vi "Programma.vi"() -> ()   [LabVIEW 2013]
panel:
  out "x = y?":bool
  in  "communicatie ?":bool=TRUE
  out "data out":string
  out "LifeForm 2":u32[][](array[colorbox])
  out "T button?":bool
  in  "Enum 2":enum16{"schrijf", "lees"}(ring)
  in  "eigen tekst":string
  in  "Eigen":bool[][](array[boolean])
  in  "Grootte":u32=20
  in  "milliseconds to wait":u32
  in  "Keuze":T1(ring)
  out "LifeForm":u32[][](array[colorbox])
  in  "Create Life uit keuze menu":bool
  # "Via keuze kan je data in de array sturen:\ninit, niks , communicatie en next versturen geen data."
  # "In het programma ( niet als server )\nAls je de eigen keuze kiest, kan je zelf iets tekenen in de eigen array OF je kan tekst tot maximum 20 tekens in de eigen tekst input typen\nDe eigen keuze geeft de optie voor het algoritme of weergeven\nAls je op weergeven duwt kan je niet switchen naar het algortime ! ( moet je het programma uitzetten en opnieuw opzetten)\nals server  via de client gaat dit wel ! ( door gewoon nieuwe data te versturen )"
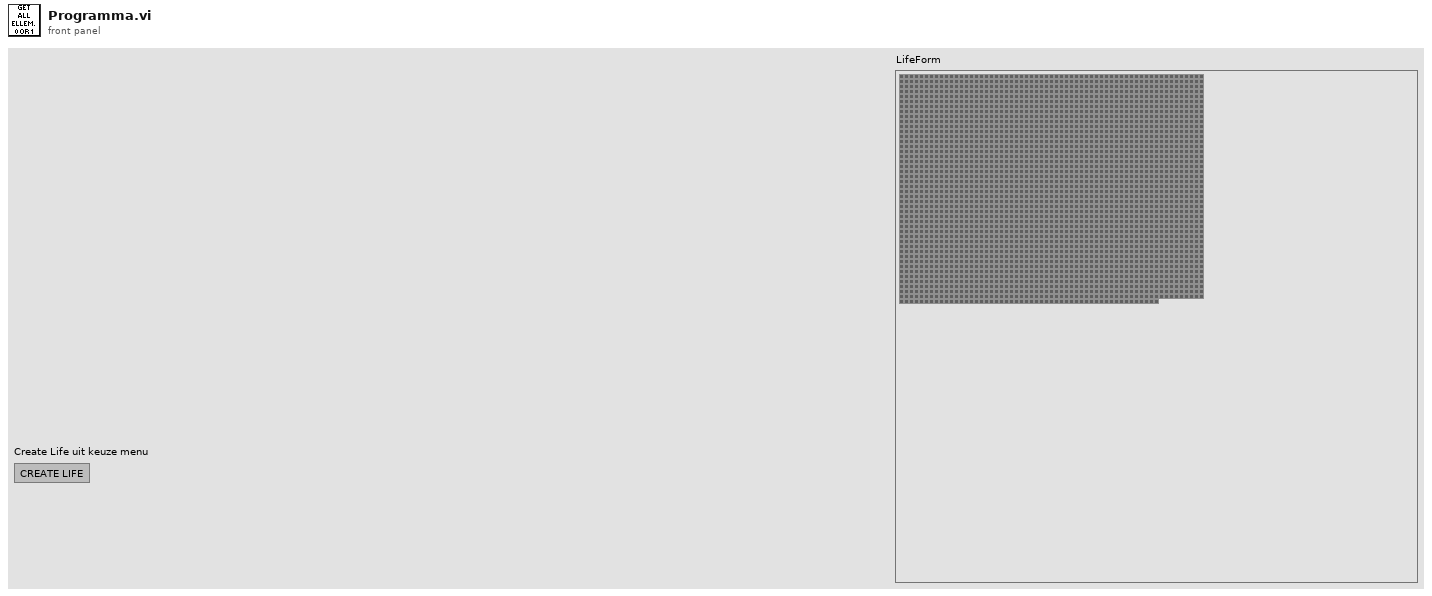
[diagram p1: front panel]
types:
  T1 = enum16{"Init", "Blinker", "Glider", "Block", "Next", "Toad", "Beehive", "Beacon", "Pulsar", "Eigen", "LWSS", "Niks", "Communicatie"}
  T2 = enum16{"Init", "Blinker", "Glider", "Block", "Next", "Toad", "Beehive", "Beacon", "Pulsar", "Eigen", "LWSS", "Niks", "Communicatie", "Lees"}
  T3 = enum16{"Init", "Blinker", "Glider", "Block", "Next"}
  T4 = enum16{"Init", "Blinker", "Glider", "Block", "Next", "Toad", "Beehive", "Beacon", "Pulsar", "Eigen", "LWSS"}
  T5 = enum16{"Init", "Blinker", "Glider", "Block", "Next", "Toad", "Beehive", "Beacon", "Pulsar", "Eigen", "LWSS", "Niks"}
  T6 = enum16{"Init", "Blinker", "Glider", "Block", "Next", "Toad"}
  T7 = enum16{"Init", "Blinker", "Glider", "Block", "Next", "Toad", "Beehive"}
  T8 = enum16{"Init", "Blinker", "Glider", "Block", "Next", "Toad", "Beehive", "Beacon"}
  T9 = enum16{"Init", "Blinker", "Glider", "Block", "Next", "Toad", "Beehive", "Beacon", "Pulsar"}
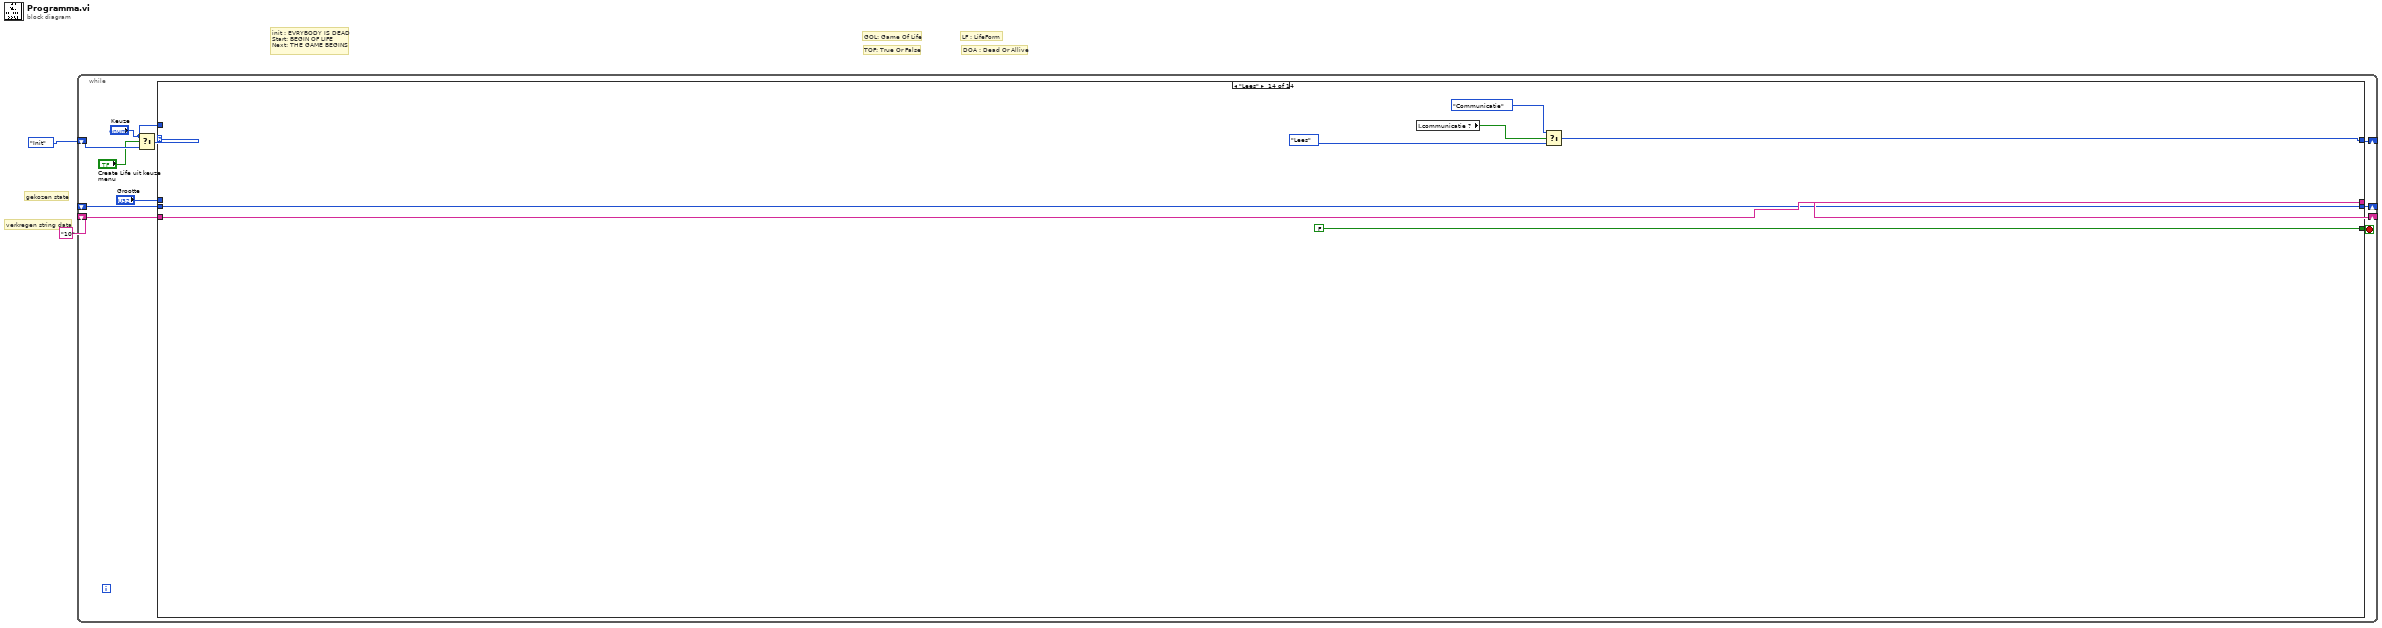
[diagram p0: block diagram]
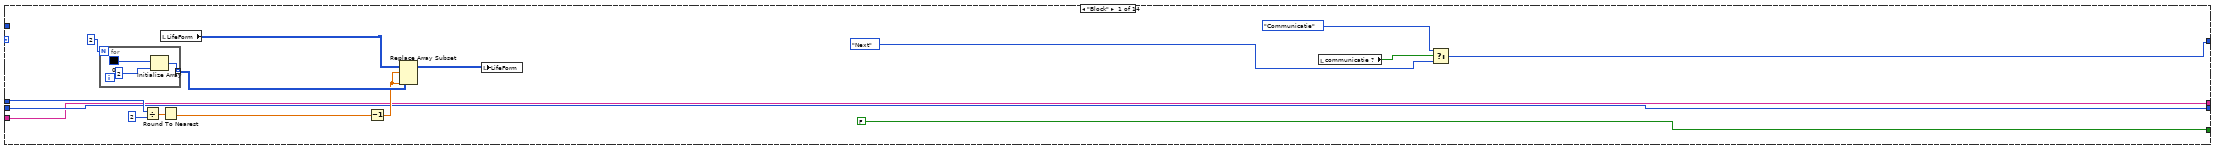
[diagram p2: hidden frame]
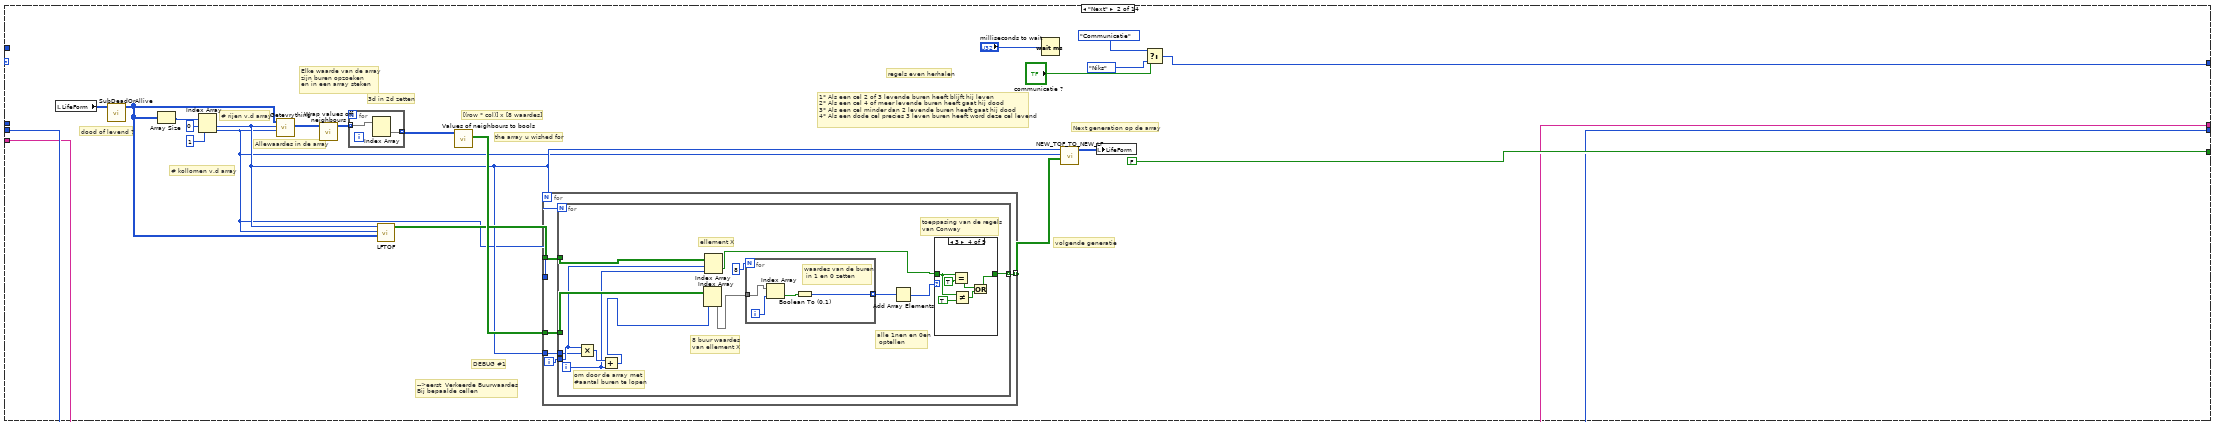
[diagram p3: hidden frame]
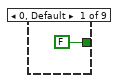
[diagram p4: hidden frame]
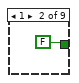
[diagram p5: hidden frame]
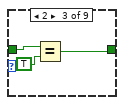
[diagram p6: hidden frame]
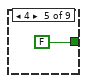
[diagram p7: hidden frame]
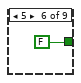
[diagram p8: hidden frame]
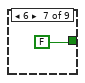
[diagram p9: hidden frame]
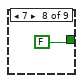
[diagram p10: hidden frame]
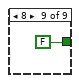
[diagram p11: hidden frame]
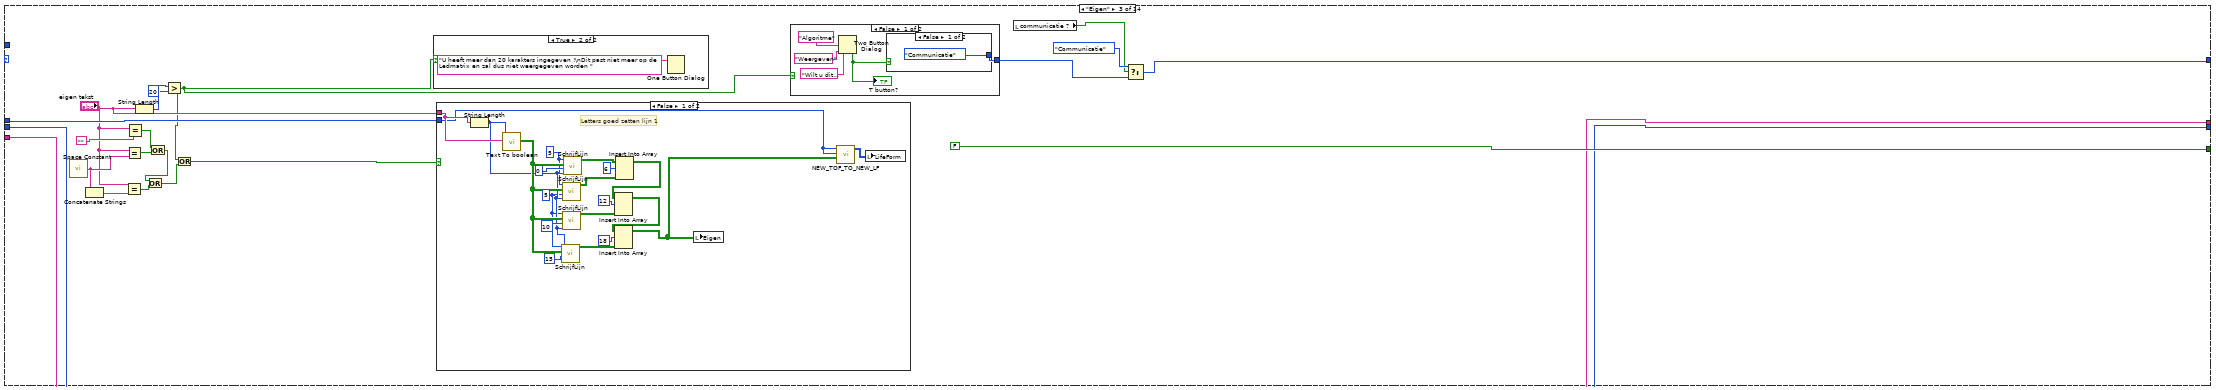
[diagram p12: hidden frame]
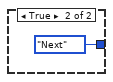
[diagram p13: hidden frame]
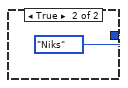
[diagram p14: hidden frame]
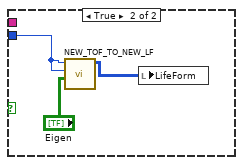
[diagram p16: hidden frame]
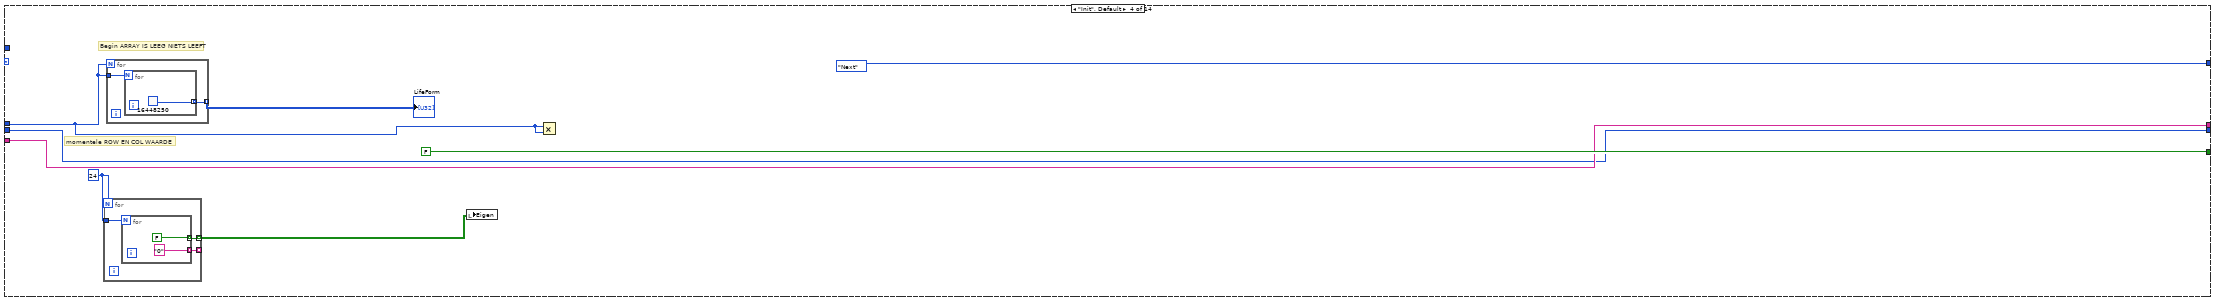
[diagram p17: hidden frame]
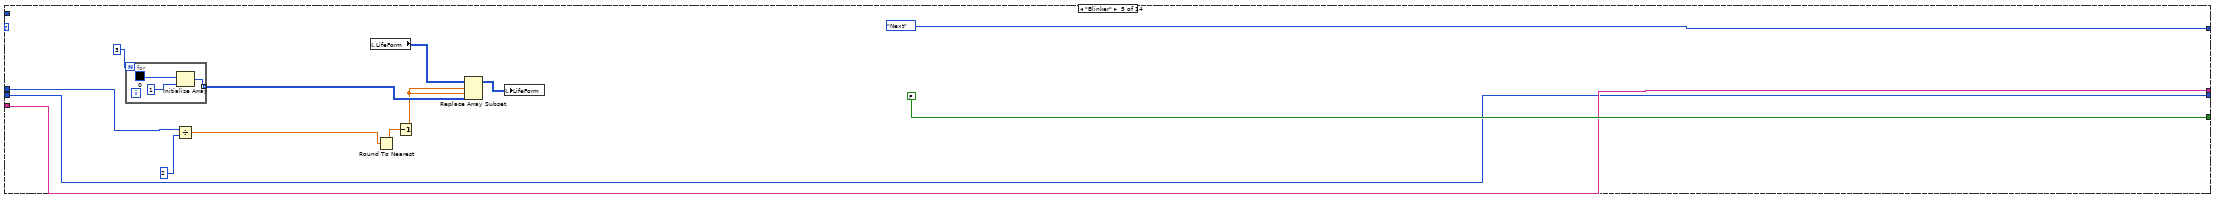
[diagram p18: hidden frame]
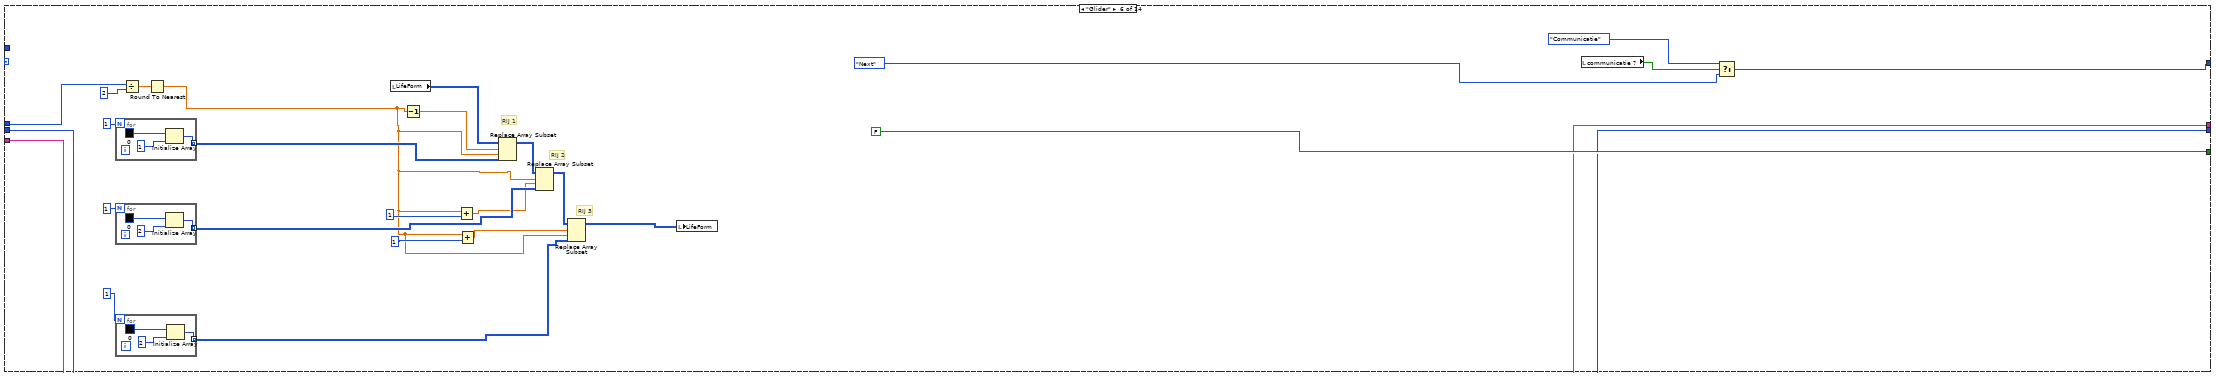
[diagram p19: hidden frame]
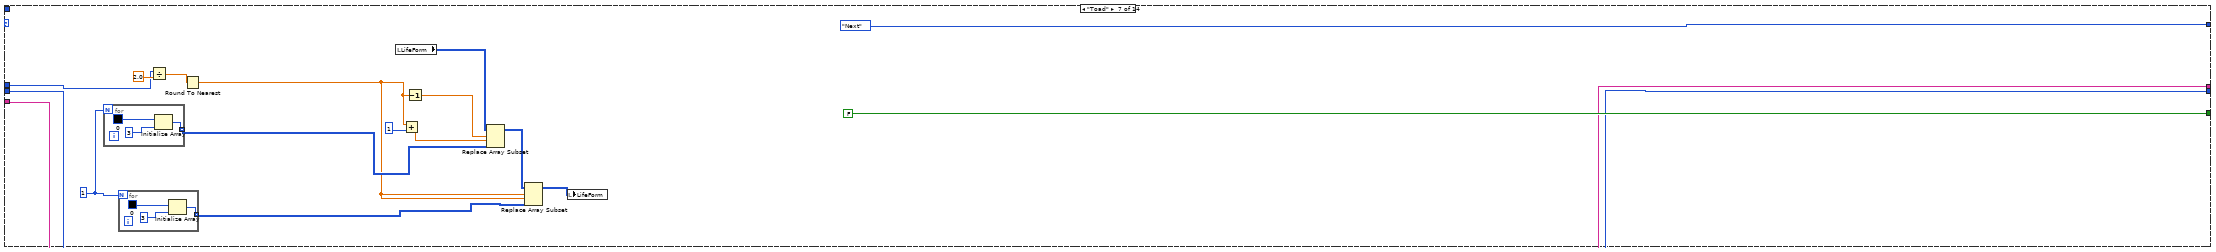
[diagram p20: hidden frame]
diagram:
  # "gekozen state"
  # "verkregen string data"
  # "DOA : Dead Or Allive"
  # "LF : LifeForm"
  # "TOF: True Or False"
  # "GOL: Game Of Life"
  # "init : EVRYBODY IS DEAD\nStart: BEGIN OF LIFE\nNext: THE GAME BEGINS"
  n1 = while {
    shift-right: [w12] -> _
    shift-left: T1."Init" ("Keuze") -> [w10]
    shift-right: [w7] -> _
    shift-left: "10" ("data out") -> [w6]
    shift-right: [w5] -> _
    shift-left: _ -> [w4]
    stop <- w13 stop-if-true
    n2 = Select(t="Keuze", s="Create Life uit keuze menu", f=w10) -> (s? t:f=w9:T2)
    n3 = case shown="\"Lees\"" w9 {
      tunnel: [FALSE FALSE FALSE FALSE FALSE FALSE FALSE FALSE FALSE FALSE FALSE FALSE w416 FALSE] -> w13
      tunnel: [w14 w38 w99 T3."Next" ("Enum") T3."Next" ("Enum") w182 T6."Next" ("Keuze") T7."Next" ("Keuze") T8."Next" ("Keuze") w284 w358 w395 w412 w497] -> w12
      tunnel: "Grootte" -> [w24 _ w116 w153 w171 w195 w225 w255 w275 w346 w371 _ w411 _]
      tunnel: "Keuze" -> [_ _ _ _ _ _ _ _ _ _ _ w400 _ _]
      tunnel: [w18 w33 w101 w150 w166 w186 w217 w240 w267 w289 w363 w402 w415 w502] -> w7
      tunnel: w6 -> [w18 w33 w101 w150 w166 w186 w217 w240 w267 w289 w363 w402 w410 w502]
      tunnel: [w19 w34 w100 w149 w165 w185 w216 w239 w266 w288 w362 w401 w412 w501] -> w5
      tunnel: w4 -> [w19 w34 w100 w149 w165 w185 w216 w239 w266 w288 w362 w401 w413 w501]
      frame "Block" {
        n4 = for {
          N: 2 -> [_]
          tunnel: [w30] -> w26 mode=indexing
          n5 = Initialize Array(u32 0 ("Color Box"), 2 ("dimension size")) -> (w30:u32[])
        }
        n6 = Divide(x=w24, y=u32 2) -> (x/y=w22:dbl)
        n7 = local read "LifeForm"() -> (w27:u32[][])
        n8 = Round To Nearest(number=w22) -> (nearest integer value=w21:dbl)
        n9 = Decrement(x=w21) -> (x-1=w20:dbl)
        n10 = Replace Array Subset(array=w27, new element=w26, index (row)=w20, index (col)=w20) -> (w25:u32[][])
        n11 = local write "LifeForm"(w25) -> ()
        n12 = local read "communicatie ?"() -> (w17:bool)
        n13 = Select(t=T2."Communicatie" ("Keuze"), s=w17, f=T3."Next" ("Enum")) -> (s? t:f=w14:T2)
      }
      frame "Next" {
        # "volgende generatie"
        # "regels even herhalen"
        # "Next generation op de array"
        # "Elke waarde van de array \nzijn buren opzoeken \nen in een array steken"
        # "-->eerst  Verkeerde Buurwaardes\nBij bepaalde cellen"
        # "dood of levend ?"
        # "Allewaardes in de array"
        # "DEBUG #1"
        # "1* Als een cel 2 of 3 levende buren heeft blijft hij leven\n2* Als een cel 4 of meer levende buren heeft gaat hij dood\n3* Als een cel minder dan 2 levende buren heeft gaat hij dood\n4* Als een dode cel precies 3 leven buren heeft word deze cel levend"
        # "[(row * col)] x [8 waardes]"
        # "# kollomen v.d array"
        # "# rijen v.d array"
        # "the array u wished for"
        # "3d in 2d zetten"
        n14 = local read "LifeForm"() -> (w44:u32[][])
        n15 = call "SubDeadOrAllive.vi"("Array"=w44) -> ("Array Dead Or Allive"=w48:u32[][])  [unwired: 10 in]
        n16 = Array Size(array=w48) -> (size(s)=w54:i32[])
        n17 = Index Array(array=w54, index #1=0 ("index"), index #2=1 ("index")) -> (element #1=w41:i32, element #2=w40:i32)
        n18 = call "Getevrything.vi"("Col"=w40, "Row"=w41, "Array Dead Or Allive"=w48) -> ("Array"=w51:u32[][][])  [unwired: 7 in, 1 out]
        n19 = call "Wrap values off neighbours.vi"("Array in"=w51) -> ("Array out"=w50:u32[][][])  [unwired: 10 in]
        n20 = for {
          tunnel: w50 -> [w95] mode=indexing
          tunnel: [w94] -> w49 mode=indexing
          n21 = Index Array(array=w95) -> (element=w94:u32[])  [unwired: 2 in]
        }
        n22 = call "LFTOF.vi"("LF DOA"=w48, "Col"=w40, "Row"=w41) -> ("LF TOF"=w46:bool[][])  [unwired: 8 in]
        n23 = call "Values of neighbours to bools.vi"("Array in"=w49) -> ("Array"=w47:bool[][])  [unwired: 9 in, 1 out]
        n24 = for {
          N: w41 -> [_]
          tunnel: w40 -> [w60]
          tunnel: w47 -> [w59]
          tunnel: w46 -> [w57]
          tunnel: [w56] -> w42 mode=indexing
          tunnel: w41 -> [w55]
          i -> [w58]
          # "om door de array met\n#aantal buren te lopen"
          n25 = for {
            N: w60 -> [_]
            tunnel: w59 -> [w73]
            tunnel: w58 -> [w68]
            tunnel: w57 -> [w70]
            tunnel: [w63] -> w56 mode=indexing
            tunnel: w55 -> [w61]
            i -> [w69]
            # "toeppasing van de regels\nvan Conway"
            # "alle 1nen en 0en\n optellen"
            # "ellement X"
            # "8 buur waardes\nvan ellement X"
            n26 = Multiply(x=w68, y=w61) -> (x*y=w72:i32)
            n27 = Add(x=w72, y=w69) -> (x+y=w71:i32)
            n28 = Index Array(array=w73, index (row)=w71) -> (element=w64:bool[])  [unwired: 1 in]
            n29 = Index Array(array=w70, index (row)=w68, index (col)=w69) -> (element=w65:bool)
            n30 = for {
              N: 8 -> [_]
              tunnel: w64 -> [w93]
              tunnel: [w90] -> w66 mode=indexing
              i -> [w92]
              # "waardes van de buren\n in 1 en 0 zetten"
              n31 = Index Array(array=w93, index=w92) -> (element=w91:bool)
              n32 = Boolean To (0,1)(Boolean=w91) -> (0, 1=w90:i16)
            }
            n33 = Add Array Elements(numeric array=w66) -> (sum=w62:i16)
            n34 = case shown="3" w62 {
              tunnel: w65 -> [_ _ w78 w83 _ _ _ _ _]
              tunnel: [FALSE FALSE w76 w79 FALSE FALSE FALSE FALSE FALSE] -> w63
              frame 0, Default {
              }
              frame 1 {
              }
              frame 2 {
                n35 = Equal?(x=w78, y=TRUE) -> (x = y?=w76:bool)
              }
              frame 3 {
                n36 = Equal?(x=w83, y=TRUE) -> (x = y?=w80:bool)
                n37 = Not Equal?(x=w83, y=TRUE) -> (x != y?=w81:bool)
                n38 = Or(x=w80, y=w81) -> (x .or. y?=w79:bool)
              }
              frame 4 {
              }
              frame 5 {
              }
              frame 6 {
              }
              frame 7 {
              }
              frame 8 {
              }
            }
          }
        }
        n39 = Wait (ms)(milliseconds to wait="milliseconds to wait") -> ()  [unwired: 1 out]
        n40 = call "NEW_TOF_TO_NEW_LF.vi"("NEXT TOF"=w42, "Col"=w40, "Row"=w41) -> ("Next LF"=w39:u32[][])  [unwired: 8 in]
        n41 = local write "LifeForm"(w39) -> ()
        n42 = Select(t=T2."Communicatie" ("Keuze"), s="communicatie ?", f=T2."Niks" ("Keuze")) -> (s? t:f=w38:T2)
      }
      frame "Eigen" {
        n43 = call <vilib>:"Space Constant.vi"() -> ("String"=w111:string)
        n44 = Concatenate Strings(w111, w111) -> (w110:string)
        n45 = Equal?(x="eigen tekst", y=w110) -> (x = y?=w109:bool)
        n46 = Equal?(x="eigen tekst", y=w111) -> (x = y?=w112:bool)
        n47 = Equal?(x="eigen tekst", y="") -> (x = y?=w113:bool)
        n48 = String Length(string="eigen tekst") -> (length=w106:i32)
        n49 = Or(x=w113, y=w112) -> (x .or. y?=w108:bool)
        n50 = Or(x=w108, y=w109) -> (x .or. y?=w104:bool)
        n51 = Greater?(x=w106, y=20) -> (0:w102:bool)
        n52 = Or(x=w102, y=w104) -> (x .or. y?=w103:bool)
        n53 = case shown="True" w102 {
          frame False {
          }
          frame True {
            n54 = One Button Dialog(message="U heeft meer dan 20 karakters ingegeven !\nDit past niet meer op de Ledmatrix en zal dus niet weergegeven worden ") -> ()  [unwired: 1 in, 1 out]
          }
        }
        n55 = case shown="False" w103 {
          tunnel: w116 -> [w144 w148]
          tunnel: "eigen tekst" -> [w145 _]
          frame False {
            w126 = 5 ("x")
            w127 = 5
            # "Letters goed zetten lijn 1"
            n56 = String Length(string=w145) -> (length=w138:i32)
            n57 = call "Text To boolean.vi"("eigen tekst"=w145, "Numeric"=w138) -> ("Letter"=w140:bool[][][])  [unwired: 9 in]
            n58 = call "SchrijfLijn.vi"("Lengte"=w138, "x"=15, "Letter in"=w140, "Numeric"=w126) -> ("Letter out"=w129:bool[][])  [unwired: 7 in]
            n59 = call "SchrijfLijn.vi"("Lengte"=w138, "x"=w126, "Letter in"=w140, "Numeric"=w127) -> ("Letter out"=w135:bool[][])  [unwired: 7 in]
            n60 = call "SchrijfLijn.vi"("Lengte"=w138, "x"=10, "Letter in"=w140, "Numeric"=w126) -> ("Letter out"=w132:bool[][])  [unwired: 7 in]
            n61 = call "SchrijfLijn.vi"("Lengte"=w138, "x"=0, "Letter in"=w140, "Numeric"=w127) -> ("Letter out"=w137:bool[][])  [unwired: 7 in]
            n62 = Insert Into Array(array=w137, index (row)=6, new element=w135) -> (w133:bool[][])  [unwired: 1 in]
            n63 = Insert Into Array(array=w133, index (row)=12, new element=w132) -> (w131:bool[][])  [unwired: 1 in]
            n64 = Insert Into Array(array=w131, index (row)=18, new element=w129) -> (w128:bool[][])  [unwired: 1 in]
            n65 = local write "Eigen"(w128) -> ()
            n66 = call "NEW_TOF_TO_NEW_LF.vi"("NEXT TOF"=w128, "Col"=w144, "Row"=w144) -> ("Next LF"=w143:u32[][])  [unwired: 8 in]
            n67 = local write "LifeForm"(w143) -> ()
          }
          frame True {
            n68 = call "NEW_TOF_TO_NEW_LF.vi"("NEXT TOF"="Eigen", "Col"=w148, "Row"=w148) -> ("Next LF"=w146:u32[][])  [unwired: 8 in]
            n69 = local write "LifeForm"(w146) -> ()
          }
        }
        n70 = case shown="False" w102 {
          tunnel: [w120 T5."Niks" ("Keuze")] -> w98
          frame False {
            n71 = Two Button Dialog(message="Wilt u dit gewoon weergeven of wilt u  het algoritme hierop toepassen ?", 1:"Weergeven" ("F button name (\"Cancel\")"), 2:"Algoritme" ("T button name (\"OK\")")) -> (T button?=w119:bool)
            "T button?" <- w119
            n72 = case shown="False" w119 {
              tunnel: [T2."Communicatie" ("Keuze") T4."Next" ("Keuze")] -> w120
              frame False {
              }
              frame True {
              }
            }
          }
          frame True {
          }
        }
        n73 = local read "communicatie ?"() -> (w96:bool)
        n74 = Select(t=T2."Communicatie" ("Keuze"), s=w96, f=w98) -> (s? t:f=w99:T2)
      }
      frame "Init", Default {
        w152 = 24
        # "momentele ROW EN COL WAARDE"
        # "Begin ARRAY IS LEEG NIETS LEEFT"
        n75 = for {
          N: w152 -> [_]
          tunnel: w152 -> [w159]
          tunnel: [w158] -> w151 mode=indexing
          tunnel: [w157] -> _ mode=indexing
          n76 = for {
            N: w159 -> [_]
            tunnel: [FALSE] -> w158 mode=indexing
            tunnel: ["0"] -> w157 mode=indexing
          }
        }
        n77 = for {
          N: w153 -> [_]
          tunnel: w153 -> [w163]
          tunnel: [w162] -> w156 mode=indexing
          n78 = for {
            N: w163 -> [_]
            tunnel: [u32 16448250 ("Color Box")] -> w162 mode=indexing
          }
        }
        "LifeForm" <- w156
        n79 = local write "Eigen"(w151) -> ()
        n80 = Multiply(x=w153, y=w153) -> ()  [unwired: 1 out]
      }
      frame "Blinker" {
        n81 = for {
          N: 3 -> [_]
          tunnel: [w178] -> w176 mode=indexing
          n82 = Initialize Array(u32 0 ("Color Box"), 1 ("dimension size")) -> (w178:u32[])
        }
        n83 = Divide(x=w171, y=u32 2) -> (x/y=w170:dbl)
        n84 = local read "LifeForm"() -> (w174:u32[][])
        n85 = Round To Nearest(number=w170) -> (nearest integer value=w168:dbl)
        n86 = Decrement(x=w168) -> (x-1=w169:dbl)
        n87 = Replace Array Subset(array=w174, new element=w176, index (row)=w169, index (col)=w169) -> (w175:u32[][])
        n88 = local write "LifeForm"(w175) -> ()
      }
      frame "Glider" {
        # "RIJ 3"
        # "RIJ 2"
        # "RIJ 1"
        n89 = for {
          N: 1 -> [_]
          tunnel: [w213] -> w201 mode=indexing
          n90 = Initialize Array(u32 0 ("Color Box"), 1 ("dimension size")) -> (w213:u32[])
        }
        n91 = for {
          N: 1 -> [_]
          tunnel: [w210] -> w199 mode=indexing
          n92 = Initialize Array(u32 0 ("Color Box"), 2 ("dimension size")) -> (w210:u32[])
        }
        n93 = for {
          N: 1 -> [_]
          tunnel: [w207] -> w197 mode=indexing
          n94 = Initialize Array(u32 0 ("Color Box"), 2 ("dimension size")) -> (w207:u32[])
        }
        n95 = Divide(x=w195, y=u32 2) -> (x/y=w189:dbl)
        n96 = Round To Nearest(number=w189) -> (nearest integer value=w187:dbl)
        n97 = local read "LifeForm"() -> (w202:u32[][])
        n98 = Decrement(x=w187) -> (x-1=w188:dbl)
        n99 = Add(x=w187, y=1 ("disabled index (col)")) -> (x+y=w193:dbl)
        n100 = Add(x=w187, y=1 ("index (row)")) -> (x+y=w190:dbl)
        n101 = Replace Array Subset(array=w202, new element=w201, index (row)=w188, index (col)=w187) -> (w200:u32[][])
        n102 = Replace Array Subset(array=w200, new element=w199, index (row)=w187, index (col)=w193) -> (w198:u32[][])
        n103 = Replace Array Subset(array=w198, new element=w197, index (row)=w190, index (col)=w187) -> (w196:u32[][])
        n104 = local write "LifeForm"(w196) -> ()
        n105 = local read "communicatie ?"() -> (w181:bool)
        n106 = Select(t=T2."Communicatie" ("Keuze"), s=w181, f=T3."Next" ("Enum")) -> (s? t:f=w182:T2)
      }
      frame "Toad" {
        w218 = 1
        n107 = for {
          N: w218 -> [_]
          tunnel: [w236] -> w224 mode=indexing
          n108 = Initialize Array(u32 0 ("Color Box"), 3 ("dimension size")) -> (w236:u32[])
        }
        n109 = for {
          N: w218 -> [_]
          tunnel: [w233] -> w231 mode=indexing
          n110 = Initialize Array(u32 0 ("Color Box"), 3 ("dimension size")) -> (w233:u32[])
        }
        n111 = Divide(x=w225, y=2.0) -> (x/y=w221:dbl)
        n112 = Round To Nearest(number=w221) -> (nearest integer value=w219:dbl)
        n113 = local read "LifeForm"() -> (w229:u32[][])
        n114 = Add(x=w219, y=1 ("disabled index (col)")) -> (x+y=w222:dbl)
        n115 = Decrement(x=w219) -> (x-1=w220:dbl)
        n116 = Replace Array Subset(array=w229, new element=w224, index (row)=w220, index (col)=w222) -> (w232:u32[][])
        n117 = Replace Array Subset(array=w232, new element=w231, index (row)=w219, index (col)=w219) -> (w230:u32[][])
        n118 = local write "LifeForm"(w230) -> ()
      }
      frame "Beehive" {
        w251 = 1
        n119 = for {
          N: w251 -> [_]
          tunnel: [w263] -> w245 mode=indexing
          n120 = Initialize Array(u32 0 ("Color Box"), 2 ("dimension size")) -> (w263:u32[])
        }
        n121 = for {
          N: w251 -> [_]
          tunnel: [w260] -> w247 mode=indexing
          n122 = Initialize Array(u32 0 ("Color Box"), 1 ("dimension size")) -> (w260:u32[])
        }
        n123 = Divide(x=w255, y=2.0) -> (x/y=w257:dbl)
        n124 = Round To Nearest(number=w257) -> (nearest integer value=w242:dbl)
        n125 = local read "LifeForm"() -> (w256:u32[][])
        n126 = Increment(x=w242) -> (x+1=w241:dbl)
        n127 = Decrement(x=w242) -> (x-1=w244:dbl)
        n128 = Replace Array Subset(array=w256, new element=w245, index (row)=w244, index (col)=w241) -> (w259:u32[][])
        n129 = Increment(x=w242) -> (x+1=w243:dbl)
        n130 = Add(x=w242, y=2.0) -> (x+y=w249:dbl)
        n131 = Replace Array Subset(array=w259, new element=w247, index (row)=w242, index (col)=w242) -> (w250:u32[][])
        n132 = Replace Array Subset(array=w250, new element=w247, index (row)=w242, index (col)=w249) -> (w246:u32[][])
        n133 = Replace Array Subset(array=w246, new element=w245, index (row)=w243, index (col)=w243) -> (w254:u32[][])
        n134 = local write "LifeForm"(w254) -> ()
      }
      frame "Beacon" {
        n135 = for {
          N: 2 -> [_]
          tunnel: [w281] -> w274 mode=indexing
          n136 = Initialize Array(u32 0 ("Color Box"), 2 ("dimension size")) -> (w281:u32[])
        }
        n137 = local read "LifeForm"() -> (w276:u32[][])
        n138 = Divide(x=w275, y=u32 2) -> (x/y=w278:dbl)
        n139 = Round To Nearest(number=w278) -> (nearest integer value=w273:dbl)
        n140 = Decrement(x=w273) -> (x-1=w277:dbl)
        n141 = Increment(x=w273) -> (x+1=w271:dbl)
        n142 = Replace Array Subset(array=w276, new element=w274, index (row)=w277, index (col)=w277) -> (w270:u32[][])
        n143 = Replace Array Subset(array=w270, new element=w274, index (row)=w271, index (col)=w271) -> (w272:u32[][])
        n144 = local write "LifeForm"(w272) -> ()
      }
      frame "Pulsar" {
        # "Horizontaal 4"
        # "VERTICAAL 2"
        # "Horizontaal 3"
        # "Horizontaal 2"
        # "Verticaal 1"
        # "Horizontaal 3"
        # "Horizontaal 1"
        n145 = for {
          N: 3 -> [_]
          tunnel: [w352] -> w301 mode=indexing
          n146 = Initialize Array(u32 0 ("Color Box"), 1 ("dimension size")) -> (w352:u32[])
        }
        n147 = for {
          N: 1 -> [_]
          tunnel: [w355] -> w294 mode=indexing
          n148 = Initialize Array(u32 0 ("Color Box"), 3 ("dimension size")) -> (w355:u32[])
        }
        n149 = Divide(x=w346, y=u32 2) -> (x/y=w348:dbl)
        n150 = Round To Nearest(number=w348) -> (nearest integer value=w291:dbl)
        n151 = local read "LifeForm"() -> (w336:u32[][])
        n152 = Subtract(x=w291, y=6.0) -> (x-y=w343:dbl)
        n153 = Add(x=w291, y=2.0) -> (x+y=w342:dbl)
        n154 = Subtract(x=w291, y=4.0) -> (x-y=w327:dbl)
        n155 = Subtract(x=w291, y=6.0) -> (x-y=w338:dbl)
        n156 = Subtract(x=w291, y=4.0) -> (x-y=w344:dbl)
        n157 = Decrement(x=w291) -> (x-1=w332:dbl)
        n158 = Increment(x=w291) -> (x+1=w330:dbl)
        n159 = Add(x=w291, y=6.0) -> (x+y=w326:dbl)
        n160 = Replace Array Subset(array=w336, new element=w294, index (row)=w343, index (col)=w344) -> (w335:u32[][])
        n161 = Replace Array Subset(array=w335, new element=w294, index (row)=w343, index (col)=w342) -> (w334:u32[][])
        n162 = Replace Array Subset(array=w334, new element=w301, index (row)=w327, index (col)=w338) -> (w333:u32[][])
        n163 = Replace Array Subset(array=w333, new element=w301, index (row)=w327, index (col)=w332) -> (w331:u32[][])
        n164 = Replace Array Subset(array=w331, new element=w301, index (row)=w327, index (col)=w330) -> (w329:u32[][])
        n165 = Replace Array Subset(array=w329, new element=w301, index (row)=w327, index (col)=w326) -> (w323:u32[][])
        n166 = Subtract(x=w291, y=6.0) -> (x-y=w307:dbl)
        n167 = Decrement(x=w291) -> (x-1=w305:dbl)
        n168 = Add(x=w291, y=6.0) -> (x+y=w302:dbl)
        n169 = Increment(x=w291) -> (x+1=w318:dbl)
        n170 = Increment(x=w291) -> (x+1=w304:dbl)
        n171 = Subtract(x=w291, y=4.0) -> (x-y=w314:dbl)
        n172 = Decrement(x=w291) -> (x-1=w319:dbl)
        n173 = Add(x=w291, y=2.0) -> (x+y=w306:dbl)
        n174 = Subtract(x=w291, y=4.0) -> (x-y=w320:dbl)
        n175 = Add(x=w291, y=2.0) -> (x+y=w322:dbl)
        n176 = Replace Array Subset(array=w323, new element=w294, index (row)=w319, index (col)=w320) -> (w321:u32[][])
        n177 = Replace Array Subset(array=w321, new element=w294, index (row)=w319, index (col)=w322) -> (w317:u32[][])
        n178 = Replace Array Subset(array=w317, new element=w294, index (row)=w318, index (col)=w314) -> (w316:u32[][])
        n179 = Replace Array Subset(array=w316, new element=w294, index (row)=w318, index (col)=w306) -> (w309:u32[][])
        n180 = Replace Array Subset(array=w309, new element=w301, index (row)=w306, index (col)=w307) -> (w312:u32[][])
        n181 = Replace Array Subset(array=w312, new element=w301, index (row)=w306, index (col)=w305) -> (w311:u32[][])
        n182 = Replace Array Subset(array=w311, new element=w301, index (row)=w306, index (col)=w304) -> (w310:u32[][])
        n183 = Replace Array Subset(array=w310, new element=w301, index (row)=w306, index (col)=w302) -> (w300:u32[][])
        n184 = Add(x=w291, y=6.0) -> (x+y=w293:dbl)
        n185 = Subtract(x=w291, y=4.0) -> (x-y=w295:dbl)
        n186 = Add(x=w291, y=2.0) -> (x+y=w290:dbl)
        n187 = Replace Array Subset(array=w300, new element=w294, index (row)=w293, index (col)=w295) -> (w298:u32[][])
        n188 = Replace Array Subset(array=w298, new element=w294, index (row)=w293, index (col)=w290) -> (w299:u32[][])
        n189 = local write "LifeForm"(w299) -> ()
        n190 = local read "communicatie ?"() -> (w285:bool)
        n191 = Select(t=T2."Communicatie" ("Keuze"), s=w285, f=T9."Next" ("Keuze")) -> (s? t:f=w284:T2)
      }
      frame "LWSS" {
        n192 = for {
          N: 1 -> [_]
          tunnel: [w389] -> w372 mode=indexing
          n193 = Initialize Array(u32 0 ("Color Box"), 4 ("dimension size")) -> (w389:u32[])
        }
        n194 = Divide(x=w371, y=u32 2) -> (x/y=w387:dbl)
        n195 = for {
          N: 1 -> [_]
          tunnel: [w392] -> w369 mode=indexing
          n196 = Initialize Array(u32 0 ("Color Box"), 2 ("dimension size")) -> (w392:u32[])
        }
        n197 = Round To Nearest(number=w387) -> (nearest integer value=w386:dbl)
        n198 = Decrement(x=w386) -> (x-1=w366:dbl)
        n199 = local read "LifeForm"() -> (w384:u32[][])
        n200 = Decrement(x=w366) -> (x-1=w365:dbl)
        n201 = Subtract(x=w366, y=2.0) -> (x-y=w380:dbl)
        n202 = Subtract(x=w366, y=2.0) -> (x-y=w374:dbl)
        n203 = Increment(x=w366) -> (x+1=w378:dbl)
        n204 = Increment(x=w366) -> (x+1=w376:dbl)
        n205 = Increment(x=w376) -> (x+1=w368:dbl)
        n206 = Increment(x=w368) -> (x+1=w367:dbl)
        n207 = Replace Array Subset(array=w384, new element=w369, index (row)=w366, index (col)=w366) -> (w382:u32[][])
        n208 = Replace Array Subset(array=w382, new element=w369, index (row)=w376, index (col)=w380) -> (w379:u32[][])
        n209 = Replace Array Subset(array=w379, new element=w369, index (row)=w376, index (col)=w378) -> (w377:u32[][])
        n210 = Replace Array Subset(array=w377, new element=w372, index (row)=w368, index (col)=w374) -> (w370:u32[][])
        n211 = Replace Array Subset(array=w370, new element=w369, index (row)=w367, index (col)=w365) -> (w364:u32[][])
        n212 = local write "LifeForm"(w364) -> ()
        n213 = local read "communicatie ?"() -> (w359:bool)
        n214 = Select(t=T2."Communicatie" ("Keuze"), s=w359, f=T4."Next" ("Keuze")) -> (s? t:f=w358:T2)
      }
      frame "Niks" {
        w396 = T2."Next" ("Keuze")
        n215 = local read "communicatie ?"() -> (w397:bool)
        n216 = Select(t=T2."Communicatie" ("Keuze"), s=w397, f=w400) -> (s? t:f=w399:T2)
        n217 = local read "T button?"() -> (w404:bool)
        n218 = Not Equal?(x=w399, y=T2."Eigen" ("Keuze")) -> (x != y?=w406:bool)
        n219 = Select(t=w396, s=w406, f=T2."Lees" ("Keuze")) -> (s? t:f=w403:T2)
        n220 = Select(t=w396, s=w404, f=w403) -> (s? t:f=w395:T2)
      }
      frame "Communicatie" {
        # "0 : kies vanuit programma\n1: block\n2: custom\n3: glider \n4: Pulsar\n5: LWSS\n6: init ( leegmaken )"
        # "An IPv4 packet is limited to a size of 65,535 bytes. However the lower layers of a TCP/IP connection typically have lower packet sizes: I.e. the \"Maximum Transmission Unit\" (MTU) for Ethernet is around 1,500 bytes.\nBandwith consideration\nBe aware that the bandwidth of a TCP/IP connection is limited. A 500,000-element array of type DBL like described in the issue above equals approximately 4MB of user data. Transferring this array three times per second already oversaturates a 100MBit/s Fast Ethernet connection."
        # "deze waardes in 1 string zetten"
        # "de hele lifeform nakijken en de waardes omzetten in 1 of 0"
        n221 = call <vilib>:"TCP Listen.vi"("port"=u16 20, "service name"="localhost") -> ("error out"=w429:errorcluster, "connection ID"=w430:refnum<k5>)  [unwired: 5 in, 3 out]
        n222 = TCP Read(connection ID=w430, bytes to read=1, error in (no error)=w429) -> (connection ID out=w423:refnum<k5>, data out=w414:string, error out=w425:errorcluster)  [unwired: 2 in]
        "data out" <- w414
        n223 = Number To Decimal String(number=w411) -> (decimal integer string=w421:string)  [unwired: 1 in]
        n224 = local read "LifeForm"() -> (w428:u32[][])
        n225 = TCP Write(connection ID=w423, data in=w421, error in (no error)=w425) -> (connection ID out=w422:refnum<k5>, error out=w424:errorcluster)  [unwired: 1 in, 1 out]
        n226 = for {
          N: w411 -> [_]
          tunnel: w428 -> [w482]
          tunnel: w411 -> [w476]
          tunnel: w422 -> [w481]
          tunnel: w424 -> [w480]
          tunnel: [w479] -> w420
          tunnel: [w478] -> w419
          i -> [w477]
          n227 = for {
            N: w476 -> [_]
            tunnel: w482 -> [w496]
            tunnel: w477 -> [w495]
            tunnel: w481 -> [w489]
            tunnel: w480 -> [w488]
            tunnel: [w487] -> w479
            tunnel: [w486] -> w478
            i -> [w484]
            # "je begint op 0 dus +1"
            # "WIT"
            n228 = Index Array(array=w496, index (row)=w495, index (col)=w484) -> (element=w494:u32)
            n229 = Equal?(x=w494, y=u32 16448250) -> (x = y?=w492:bool)
            n230 = Select(t=0.0, s=w492, f=1.0) -> (s? t:f=w490:dbl)
            n231 = Number To Decimal String(number=w490) -> (decimal integer string=w483:string)  [unwired: 1 in]
            n232 = TCP Write(connection ID=w489, data in=w483, error in (no error)=w488) -> (connection ID out=w487:refnum<k5>, error out=w486:errorcluster)  [unwired: 1 in, 1 out]
          }
        }
        n233 = case shown="No Error" w419 {
          tunnel: w420 -> [w474 _]
          tunnel: w419 -> [w473 _]
          tunnel: [FALSE ("abort (F)") TRUE ("abort (F)")] -> w417
          frame No Error {
            n234 = TCP Close Connection(connection ID=w474, error in (no error)=w473) -> ()  [unwired: 1 in, 2 out]
          }
          frame Error {
          }
        }
        n235 = Equal?(x=w414, y=w410) -> (x = y?=w409:bool)
        "x = y?" <- w409
        n236 = case shown="True" w409 {
          selector: w409 -> [w433 _]
          tunnel: [w432 w455] -> w412
          tunnel: [w434 w456] -> w415
          tunnel: w414 -> [w435 w456]
          tunnel: w413 -> [_ w457]
          frame False {
            n237 = case shown="\"7\"" w435 {
              selector: w435 -> [w436 w439 w440 w442 w445 w446 w449 w450]
              tunnel: [T2."Block" ("Keuze") T2."Eigen" ("Keuze") T2."Glider" ("Keuze") T2."Pulsar" ("Keuze") T2."LWSS" ("Keuze") T2."Init" ("Keuze") T2."Niks" ("Keuze") w451] -> w432
              tunnel: [w436 w439 w440 w442 w445 w446 w449 w450] -> w434
              tunnel: w433 -> [_ _ _ _ _ _ _ _]
              frame "1" {
              }
              frame "2" {
              }
              frame "3" {
              }
              frame "4" {
              }
              frame "5" {
              }
              frame "6" {
                # "Begin ARRAY IS LEEG NIETS LEEFT"
              }
              frame "0", Default {
              }
              frame "7" {
                n238 = local read "T button?"() -> (w454:bool)
                n239 = Select(t=T2."Niks" ("Keuze"), s=w454, f=T2."Lees" ("Keuze")) -> (s? t:f=w451:T2)
              }
            }
          }
          frame True {
            n240 = case shown="\"1\", Default" w456 {
              tunnel: w457 -> [_ _ _ _ _ _ _ _]
              tunnel: [T2."Niks" ("Keuze") T2."Niks" ("Keuze") w463 T2."Niks" ("Keuze") T2."Niks" ("Keuze") T2."Niks" ("Keuze") T2."Niks" ("Keuze") w468] -> w455
              frame "1", Default {
              }
              frame "0" {
              }
              frame "2" {
                n241 = local read "T button?"() -> (w462:bool)
                n242 = Select(t=T2."Niks" ("Keuze"), s=w462, f=T2."Lees" ("Keuze")) -> (s? t:f=w463:T2)
              }
              frame "3" {
              }
              frame "4" {
              }
              frame "5" {
              }
              frame "6" {
              }
              frame "7" {
                n243 = local read "T button?"() -> (w471:bool)
                n244 = Select(t=T2."Niks" ("Keuze"), s=w471, f=T2."Lees" ("Keuze")) -> (s? t:f=w468:T2)
              }
            }
          }
        }
        n245 = Or(x=FALSE, y=w417) -> (x .or. y?=w416:bool)
      }
      frame "Lees" {
        n246 = local read "communicatie ?"() -> (w499:bool)
        n247 = Select(t=T2."Communicatie" ("Keuze"), s=w499, f=T2."Lees" ("Keuze")) -> (s? t:f=w497:T2)
      }
    }
  }
